vi "Check_over_timer.vi"(0 "Lavatory TImer":timestamp, 5 "Time Now":timestamp, 7 "Limit":i32) -> (4 "Trigger":bool)   [LabVIEW 2023, in "Lavatory_Management.lvlib"]
doc: "Check if the timer value is greater than the limit"
uses:
  Lavatory_Management.lvlib
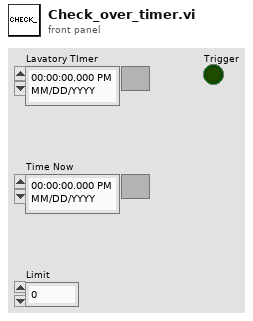
[diagram p1: front panel]
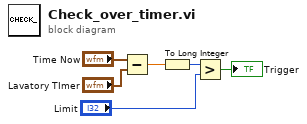
[diagram p0: block diagram]
diagram:
  n1 = Subtract(x="Time Now", y="Lavatory TImer") -> (x-y=w6:dbl)
  n2 = To Long Integer(number=w6) -> (32bit integer=w3:i32)
  n3 = Greater?(x=w3, y="Limit") -> (0:→"Trigger":bool)
